vi "NetComm_getJoystickDesc.vi"(8 "error in (no error)":errorcluster, 11 "Joystick Number":i32) -> (0 "error out":errorcluster, 2 "Axis Types":u8[](array[numeric]), 3 "Name":string, 4 "POV Count":u8, 5 "Type":u8, 6 "Button Count":u8, 7 "Is XBox":bool)   [LabVIEW 2017]
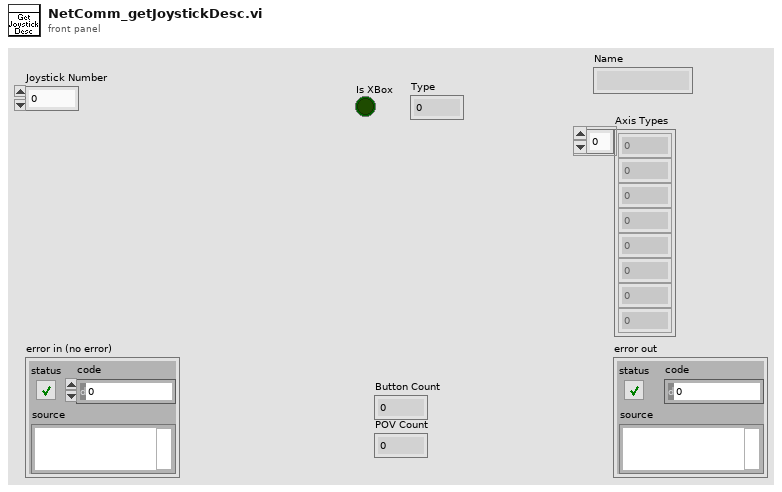
[diagram p1: front panel]
types:
  T1 = enum16{"big-endian, network order", "native, host order", "little-endian"}
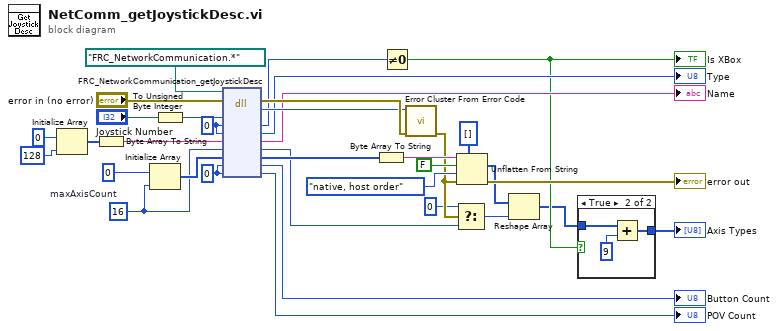
[diagram p0: block diagram]
diagram:
  w5 = u8 0 ("isXBox")
  w4 = u8 0 ("povCount")
  w20 = u8 16  # maxAxisCount
  n1 = Initialize Array(u8 0, 128 ("dimension size")) -> (w19:u8[])
  n2 = Byte Array To String(unsigned byte array=w19) -> (string=w16:string)
  n3 = Initialize Array(u8 0, w20) -> (w21:u8[])
  n4 = To Unsigned Byte Integer(number="Joystick Number") -> (unsigned 8bit integer=w22:u8)
  n5 = dll-call lib="?" fn="FRC_NetworkCommunication_getJoystickDesc"(path in=path "FRC_NetworkCommunication.*", error in="error in (no error)", "joystickNum"=w22, "isXBox"=w5, "type"=w5, "name"=w16, "axisCount"=w20, "axisTypes"=w21, "buttonCount"=w4, "povCount"=w4) -> (error out=w24:errorcluster, "return type"=w23:i32, "isXBox"=w12:u8, "type"=→"Type":u8, "name"=→"Name":string, "axisCount"=w8:u8, "axisTypes"=w15:u8[], "buttonCount"=→"Button Count":u8, "povCount"=→"POV Count":u8)  [unwired: 2 in, 1 out]
  n6 = Byte Array To String(unsigned byte array=w15) -> (string=w31:string)
  n7 = Not Equal To 0?(x=w12) -> (x != 0?=w3:bool)
  "Is XBox" <- w3
  n8 = call <vilib>:"Error Cluster From Error Code.vi"("error in (no error)"=w24, "error code (0)"=w23) -> ("error out"=w9:errorcluster)  [unwired: 7 in]
  n9 = Select(t=u8 0, s=w9, f=w8) -> (s? t:f=w7:u8)
  n10 = Unflatten From String(type=u8[] [], binary string=w31, data includes array or string size? (T)=FALSE, byte order (0:big-endian, network order)=T1."native, host order", error in (no error)=w9) -> (value=w27:u8[], error out=→"error out":errorcluster)  [unwired: 1 out]
  n11 = Reshape Array(w27, w7) -> (w2:u8[])
  n12 = case shown="True" w3 {
    tunnel: w2 -> [w35 w38]
    tunnel: [w35 w37] -> w1
    frame False {
    }
    frame True {
      n13 = Add(x=w38, y=u8 9) -> (x+y=w37:u8[])
    }
  }
  "Axis Types" <- w1
